vi "HIOKI PW3390 Conf CH A DC.vi"(0 "VISA Resource":refnum<visa-resource-name>, 1 "Set/Query (F: Set)":bool, 5 "Range (1: 5V)":enum16{"1", "5", "10"}(ring)=enum."5", 7 "Scaling (1.00)":dbl=1.0 min=0.01 max=9999.99 format="%.2f", 9 "Unit (3: Nm)":enum16{"V", "Hz", "mNm", "Nm", "kNm"}(ring)=enum."Nm", 11 "error in (no error)":errorcluster, 12 "OPC query (T: ON)":bool=TRUE, 13 "Error Out (F: Off)":bool) -> (3 "CH A input out":enum16{"FREQ", "DC"}(ring)=enum."DC", 4 "VISA Resource out":refnum<visa-resource-name>, 6 "Range out":enum16{"1", "5", "10"}(ring)=enum."5", 8 "Scaling out":dbl=1.0 format="%.2f", 10 "Unit out":enum16{"V", "Hz", "mNm", "Nm", "kNm"}(ring)=enum."Nm", 15 "error out":errorcluster)   [LabVIEW 2009]
doc: "Sets and reads the function related to the Motor Analysis Option's Channel A voltage.\n\nSet/Query\n Set: Send the setting commands for the device.\n Query: Query the setting of the device.\n\nRange\n Sets the voltage range of Channel A.\n\nScaling\n Sets the scaling of Channel A. \n Input Range: 0. 01 - 9999.99\n\nUnit\n Sets the Channel A unit."
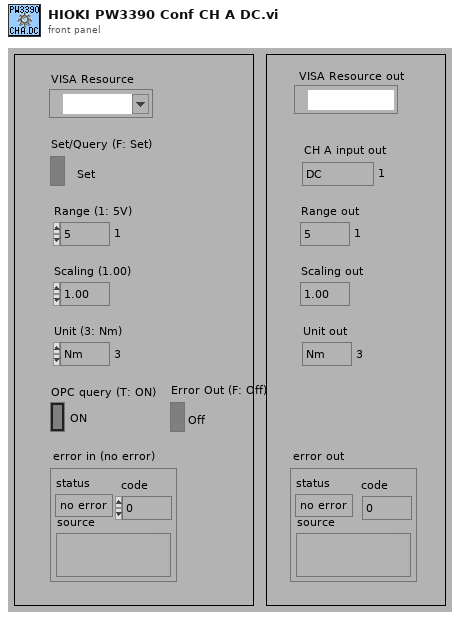
[diagram p1: front panel]
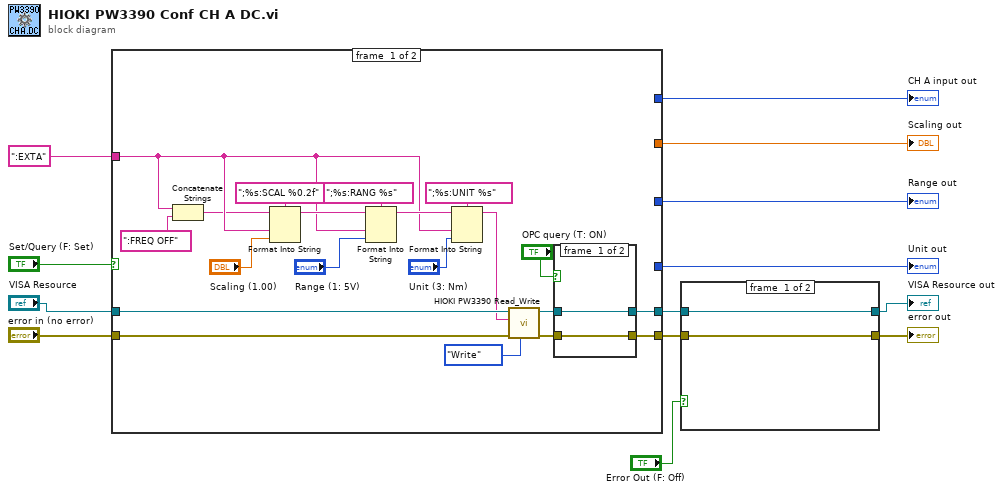
[diagram p0: block diagram]
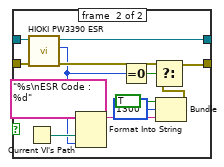
[diagram p2: hidden frame]
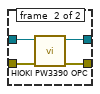
[diagram p3: hidden frame]
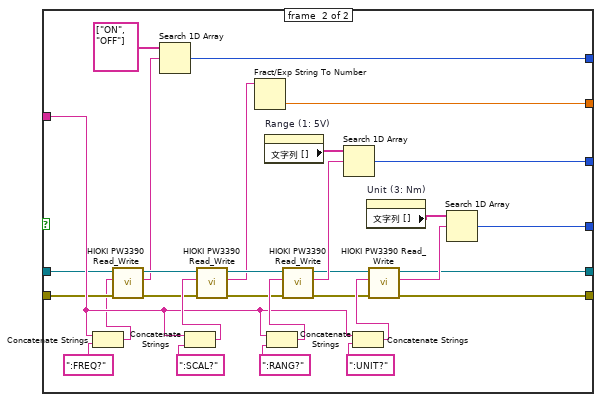
[diagram p4: hidden frame]
diagram:
  n1 = case shown="FALSE" "Set/Query (F: Set)" {
    tunnel: "error in (no error)" -> [w30 w47]
    tunnel: [w18 w57] -> w5
    tunnel: "VISA Resource" -> [w31 w48]
    tunnel: [w19 w58] -> w6
    tunnel: [_ w56] -> w11
    tunnel: ":EXTA" -> [w16 w49]
    tunnel: [_ w52] -> w9
    tunnel: [_ w66] -> w8
    tunnel: [_ w40] -> w1
    frame #0 {
      n2 = Concatenate Strings(w16, ":FREQ OFF") -> (w15:string)
      n3 = Format Into String(format string=";%s:SCAL %0.2f", initial string=w15, w16, "Scaling (1.00)") -> (resulting string=w27:string)  [unwired: 1 in, 1 out]
      n4 = Format Into String(format string=";%s:RANG %s", initial string=w27, w16, "Range (1: 5V)") -> (resulting string=w17:string)  [unwired: 1 in, 1 out]
      n5 = Format Into String(format string=";%s:UNIT %s", initial string=w17, w16, "Unit (3: Nm)") -> (resulting string=w25:string)  [unwired: 1 in, 1 out]
      n6 = call <instrlib>:"HIOKI PW3390 Read_Write.vi"("Read/Write"=enum16{"Read", "Write"}."Write", "error in (no error)"=w30, "data in"=w25, "VISA Resource"=w31) -> ("error out"=w20:errorcluster, "VISA Resource out"=w21:refnum<visa-resource-name>)  [unwired: 5 in, 1 out]
      n7 = case shown="TRUE" "OPC query (T: ON)" {
        tunnel: [w35 w39] -> w19
        tunnel: [w34 w38] -> w18
        tunnel: w21 -> [w35 w37]
        tunnel: w20 -> [w34 w36]
        frame #0 {
        }
        frame #1 {
          n8 = call <instrlib>:"HIOKI PW3390 OPC.vi"("error in (no error)"=w36, "VISA Resource"=w37) -> ("error out"=w38:errorcluster, "VISA Resource out"=w39:refnum<visa-resource-name>)  [unwired: 7 in, 1 out]
        }
      }
    }
    frame #1 {
      n9 = Concatenate Strings(w49, ":FREQ?" ("文字列")) -> (w43:string)
      n10 = call <instrlib>:"HIOKI PW3390 Read_Write.vi"("error in (no error)"=w47, "data in"=w43, "VISA Resource"=w48) -> ("error out"=w45:errorcluster, "data out"=w41:string, "VISA Resource out"=w46:refnum<visa-resource-name>)  [unwired: 6 in]
      n11 = Search 1D Array(1D array=string[] ["ON", "OFF"] ("文字列配列"), element=w41) -> (index of element=w40:i32)  [unwired: 1 in]
      n12 = Concatenate Strings(w49, ":SCAL?") -> (w61:string)
      n13 = call <instrlib>:"HIOKI PW3390 Read_Write.vi"("error in (no error)"=w45, "data in"=w61, "VISA Resource"=w46) -> ("error out"=w63:errorcluster, "data out"=w55:string, "VISA Resource out"=w64:refnum<visa-resource-name>)  [unwired: 6 in]
      n14 = Fract/Exp String To Number(string=w55) -> (number=w56:dbl)  [unwired: 3 in, 1 out]
      n15 = property on="Range (1: 5V)" class="Enum (strict)"() -> ("文字列 []"=w54:string[])  [unwired: 2 in, 2 out]
      n16 = Concatenate Strings(w49, ":RANG?") -> (w65:string)
      n17 = call <instrlib>:"HIOKI PW3390 Read_Write.vi"("error in (no error)"=w63, "data in"=w65, "VISA Resource"=w64) -> ("error out"=w50:errorcluster, "data out"=w53:string, "VISA Resource out"=w51:refnum<visa-resource-name>)  [unwired: 6 in]
      n18 = Search 1D Array(1D array=w54, element=w53) -> (index of element=w52:i32)  [unwired: 1 in]
      n19 = Concatenate Strings(w49, ":UNIT?") -> (w62:string)
      n20 = property on="Unit (3: Nm)" class="Enum (strict)"() -> ("文字列 []"=w60:string[])  [unwired: 2 in, 2 out]
      n21 = call <instrlib>:"HIOKI PW3390 Read_Write.vi"("error in (no error)"=w50, "data in"=w62, "VISA Resource"=w51) -> ("error out"=w57:errorcluster, "data out"=w59:string, "VISA Resource out"=w58:refnum<visa-resource-name>)  [unwired: 6 in]
      n22 = Search 1D Array(1D array=w60, element=w59) -> (index of element=w66:i32)  [unwired: 1 in]
    }
  }
  "Scaling out" <- w11
  "Unit out" <- w8
  "Range out" <- w9
  "CH A input out" <- w1
  n23 = case shown="TRUE" "Error Out (F: Off)" {
    tunnel: w6 -> [w71 w84]
    tunnel: w5 -> [w70 w83]
    tunnel: [w70 w73] -> w4
    tunnel: [w71 w82] -> w2
    frame #0 {
    }
    frame #1 {
      n24 = Current VI's Path() -> (path=w80:path)
      n25 = call <instrlib>:"HIOKI PW3390 ESR.vi"("error in (no error)"=w83, "VISA Resource"=w84) -> ("error out"=w74:errorcluster, "Output Value"=w72:u8, "VISA Resource out"=w82:refnum<visa-resource-name>)  [unwired: 6 in, 1 out]
      n26 = Format Into String(format string="%s\nESR Code : %d", w80, w72) -> (resulting string=w76:string)  [unwired: 2 in, 1 out]
      n27 = Equal To 0?(x=w72) -> (x = 0?=w81:bool)
      n28 = Bundle("status"=TRUE, "code"=1300, w76) -> (w75:cluster{"status":bool, "code":i32, string})  [unwired: 1 in]
      n29 = Select(t=w74, s=w81, f=w75) -> (s? t:f=w73:errorcluster)
    }
  }
  "error out" <- w4
  "VISA Resource out" <- w2
